vi "Reinterpret I16 as U16.vi"(7 "Input":i16) -> (8 "Output":u16)   [LabVIEW 2012]
uses:
  <vilib>/rvi/FXPMathLib/FxpInterpret/XNode/nifxpmath_Interpret.xnode
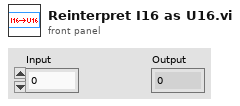
[diagram p1: front panel]
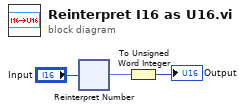
[diagram p0: block diagram]
diagram:
  n1 = xnode "Reinterpret Number"("x"="Input") -> ("y"=w3:fxp<+/-,16,16>)
  n2 = To Unsigned Word Integer(number=w3) -> (unsigned 16bit integer=→"Output":u16)
